vi "Cleanup.vi"(8 "error in (no error)":errorcluster, 11 "UIMessage in":refnum<class "UIMessage.lvclass">) -> (0 "error out":errorcluster)   [LabVIEW 2020, in "TSS.lvlib" / "UIMessage.lvclass"]
uses:
  UIMessage.lvclass
  UIMessage.lvclass/UIMessage.ctl
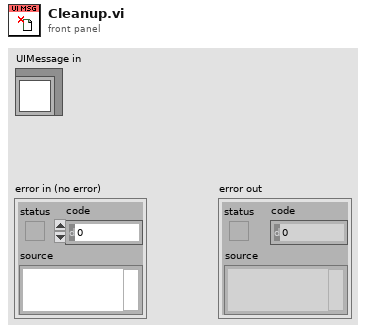
[diagram p1: front panel]
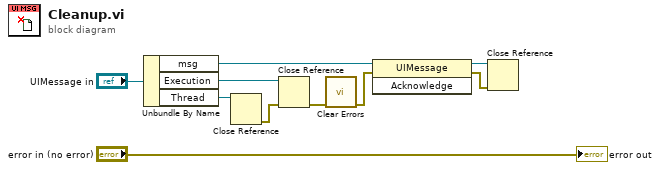
[diagram p0: block diagram]
diagram:
  n1 = Unbundle By Name("UIMessage in") -> ("msg"=w4:refnum<k7>, "Execution"=w7:refnum<k7>, "Thread"=w8:refnum<k7>)
  n2 = Close Reference(reference=w8) -> (error out=w6:errorcluster)  [unwired: 1 in]
  n3 = Close Reference(reference=w7, error in (no error)=w6) -> (error out=w5:errorcluster)
  n4 = call <vilib>:"Clear Errors.vi"("error in (no error)"=w5) -> ("error out"=w3:errorcluster)  [unwired: 5 in, 1 out]
  n5 = invoke class="UIMessage" method="Acknowledge"(reference=w4, error in=w3) -> (reference out=w1:refnum<k7>, error out=w2:errorcluster)  [unwired: 1 in, 1 out]
  n6 = Close Reference(reference=w1, error in (no error)=w2) -> ()  [unwired: 1 out]
  "error out" <- "error in (no error)"
